vi "CursorShow.vi"(7 "nameShow":bool, 8 "错误输入（无错误）":errorcluster, 9 "游标.游标位置":T1, 10 "Type":T3 caption="事件类型", 11 "Graph":refnum<vi>) -> (0 "错误输出":errorcluster, 3 "引用输出":refnum<vi>)   [LabVIEW 2020]
uses:
  <vilib>/event_ctls.llb/lveventtype.ctl
  <vilib>/Utility/miscctls.llb/LVCursorListTypeDef.ctl
  <vilib>/Utility/miscctls.llb/LVPointDoubleTypeDef.ctl
panel:
  in  "游标列表":T2=[{"Name"="游标0", "Color"=16776960, "Style"=8, "Point Style"=13, "Name Visible"=TRUE, "Allow Drag"=TRUE, "Cursor Mode"=0, "Plot"=0, "Index"=0, "Position"={"X"=0.0, "Y"=0.0}, "X Scale"=0, "Y Scale"=0, "Watch Plots"=[], "Watch All Plots"=FALSE, "Plot Area"=0, "Label Offset"={"X"=0.0, "Y"=2.8391167192429023}}]
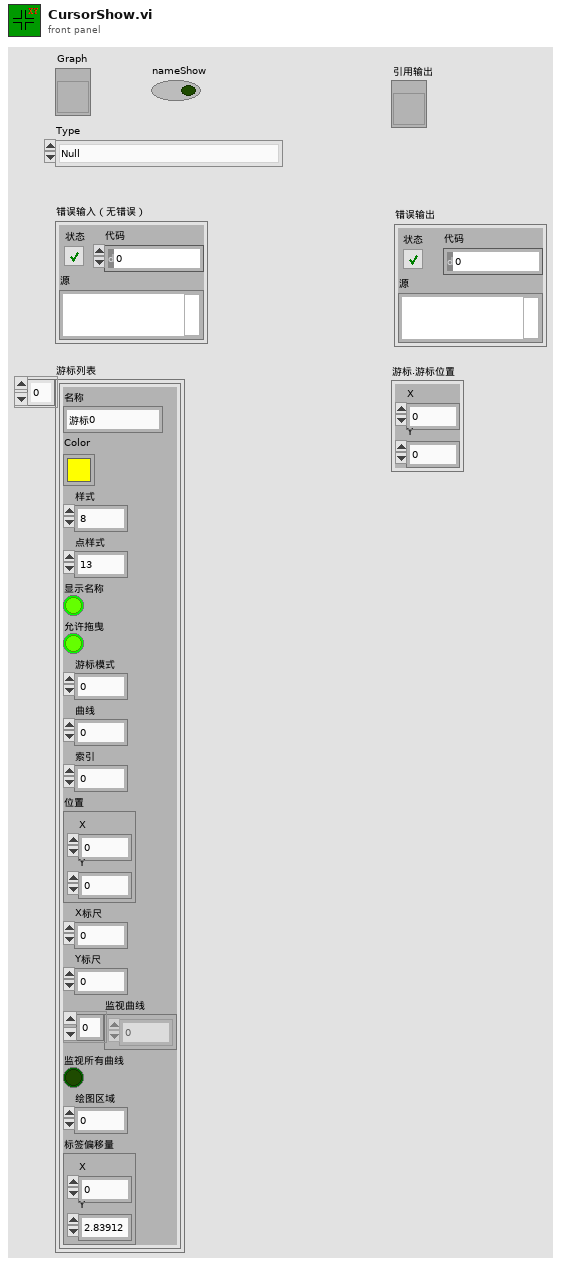
[diagram p1: front panel]
types:
  T1 = typedef "LVPointDoubleTypeDef.ctl" = cluster{"X":dbl, "Y":dbl}
  T2 = typedef "LVCursorListTypeDef.ctl" = cluster{"Name":string, "Color":u32, "Style":u8, "Point Style":u8, "Name Visible":bool, "Allow Drag":bool, "Cursor Mode":u32, "Plot":i32, "Index":i32, "Position":cluster{"X":dbl, "Y":dbl}, "X Scale":u32, "Y Scale":u32, "Watch Plots":i32[], "Watch All Plots":bool, "Plot Area":i32, "Label Offset":cluster{"X":dbl, "Y":dbl}}[]
  T3 = typedef "lveventtype.ctl" = enum32{"Null", "Timeout", "Annotation Menu Selection", "Annotation Menu Selection?", "App Instance Close", "App Instance Close?", "Autoscale Range Change", "Bookmark Info Change", "Cell Edit", "Cell Edit?", "Cursor Grab", "Cursor Grab?", "Cursor Menu Selection", "Cursor Menu Selection?", "Cursor Move", "Cursor Release", "Data Change", "Direction Change", "Display State Change", "Drag Ended", "Drag Enter", "Drag Leave", "Drag Over", "Drag Source Update", "Drag Starting", "Drag Starting?", "Drop", "Exec State Change", "Key Down", "Key Down?", "Key Repeat", "Key Repeat?", "Key Up", "Listbox Double Click", "Menu Activation?", "Menu Selection (App)", "Menu Selection? (App)", "Menu Selection (User)", "Mouse Down", "Mouse Down?", "Mouse Enter", "Mouse Leave", "Mouse Move", "Mouse Up", "Mouse Wheel", "NI Security User Change (App)", "Pane Size", "Panel Close", "Panel Close?", "Panel Resize", "Plot Attribute Change", "Scale Range Change", "Shortcut Menu Activation?", "Shortcut Menu Selection (App)", "Shortcut Menu Selection? (App)", "Shortcut Menu Selection (User)", "Tree Double Click", "Tree Drag", "Tree Drag?", "Tree Drop", "Tree Drop?", "Tree Item Close", "Tree Item Close?", "Tree Item Open", "Tree Item Open?", "User Event", "Value Change"}
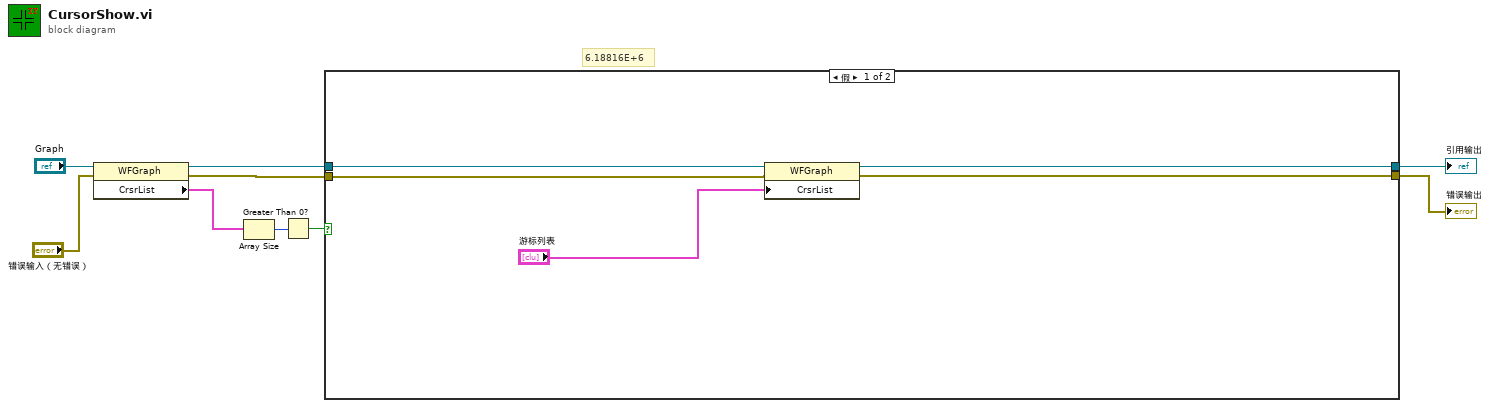
[diagram p0: block diagram]
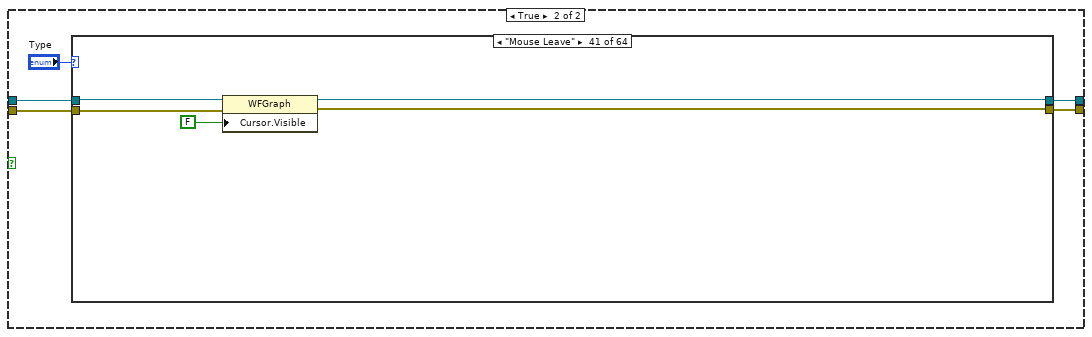
[diagram p2: hidden frame]
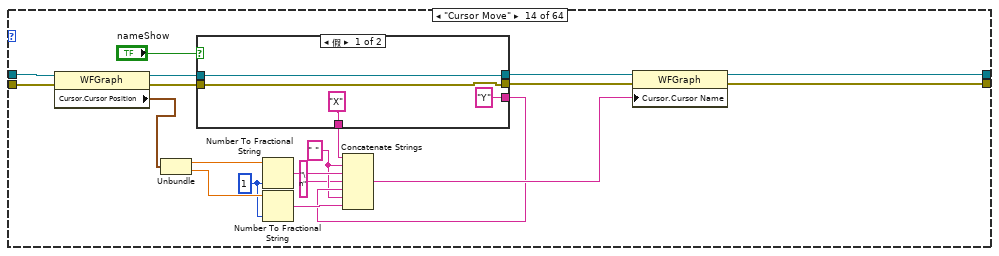
[diagram p16: hidden frame]
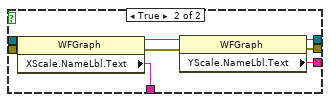
[diagram p17: hidden frame]
diagram:
  # "6.18816E+6"
  n1 = property class="WFGraph"(reference="Graph", error in="错误输入（无错误）") -> (reference out=w5:refnum<vi>, error out=w3:errorcluster, "CrsrList"=w8:T2)
  n2 = Array Size(array=w8) -> (size(s)=w9:i32)
  n3 = Greater Than 0?(x=w9) -> (x > 0?=w7:bool)
  n4 = case shown="假" w7 {
    tunnel: w5 -> [w14 w19]
    tunnel: w3 -> [w11 w17]
    tunnel: [w12 w16] -> w2
    tunnel: [w13 w15] -> w1
    frame False {
      n5 = property class="WFGraph"(reference=w14, error in=w11, "CrsrList"="游标列表") -> (reference out=w13:refnum<vi>, error out=w12:errorcluster)
    }
    frame True {
      n6 = case shown="\"Mouse Leave\"" "Type" {
        tunnel: w19 -> [_ _ _ _ _ _ _ _ _ _ _ _ _ w39 _ _ _ _ _ _ _ _ _ _ _ _ _ _ _ _ _ _ _ _ _ _ _ w54 _ w59 w66 _ _ _ _ _ _ _ _ _ _ _ _ _ _ _ _ _ _ _ _ _ _ _]
        tunnel: w17 -> [_ _ _ _ _ _ _ _ _ _ _ _ _ w25 _ _ _ _ _ _ _ _ _ _ _ _ _ _ _ _ _ _ _ _ _ _ _ _ _ w58 w64 _ _ _ _ _ _ _ _ _ _ _ _ _ _ _ _ _ _ _ _ _ _ _]
        tunnel: [_ _ _ _ _ _ _ _ _ _ _ _ _ w22 _ _ _ _ _ _ _ _ _ _ _ _ _ _ _ _ _ _ _ _ _ _ _ _ _ w56 w63 _ _ _ _ _ _ _ _ _ _ _ _ _ _ _ _ _ _ _ _ _ _ _] -> w16
        tunnel: [_ _ _ _ _ _ _ _ _ _ _ _ _ w21 _ _ _ _ _ _ _ _ _ _ _ _ _ _ _ _ _ _ _ _ _ _ _ w53 _ w55 w62 _ _ _ _ _ _ _ _ _ _ _ _ _ _ _ _ _ _ _ _ _ _ _] -> w15
        frame "Null", Default {
        }
        frame "Timeout" {
        }
        frame "Annotation Menu Selection" {
        }
        frame "Annotation Menu Selection?" {
        }
        frame "App Instance Close" {
        }
        frame "App Instance Close?" {
        }
        frame "Autoscale Range Change" {
        }
        frame "Cell Edit" {
        }
        frame "Cell Edit?" {
        }
        frame "Cursor Grab" {
        }
        frame "Cursor Grab?" {
        }
        frame "Cursor Menu Selection" {
        }
        frame "Cursor Menu Selection?" {
        }
        frame "Cursor Move" {
          w27 = " " ("字符串")
          w36 = i16 1 ("精度(6)")
          n7 = property class="WFGraph"(reference=w39, error in=w25) -> (reference out=w32:refnum<vi>, error out=w24:errorcluster, "Cursor.Cursor Position"=w34:T1)
          n8 = Unbundle(w34) -> ("Cursor X"=w38:dbl, "Cursor Y"=w37:dbl)
          n9 = case shown="假" "nameShow" {
            tunnel: w32 -> [w41 w51]
            tunnel: [w41 w49] -> w31
            tunnel: ["X" ("XScale.NameLbl.Text") w48] -> w30
            tunnel: ["Y" ("YScale.NameLbl.Text") w47] -> w28
            tunnel: w24 -> [w40 w46]
            tunnel: [w40 w44] -> w23
            frame False {
            }
            frame True {
              n10 = property class="WFGraph"(reference=w51, error in=w46) -> (reference out=w50:refnum<vi>, error out=w45:errorcluster, "XScale.NameLbl.Text"=w48:string)
              n11 = property class="WFGraph"(reference=w50, error in=w45) -> (reference out=w49:refnum<vi>, error out=w44:errorcluster, "YScale.NameLbl.Text"=w47:string)
            }
          }
          n12 = Number To Fractional String(number=w38, precision (6)=w36) -> (F-format string=w35:string)  [unwired: 2 in]
          n13 = Number To Fractional String(number=w37, precision (6)=w36) -> (F-format string=w29:string)  [unwired: 2 in]
          n14 = Concatenate Strings(w30, w27, w35, "\n" ("字符串"), w28, w27, w29) -> (w33:string)
          n15 = property class="WFGraph"(reference=w31, error in=w23, "Cursor.Cursor Name"=w33) -> (reference out=w21:refnum<vi>, error out=w22:errorcluster)
        }
        frame "Cursor Release" {
        }
        frame "Data Change" {
        }
        frame "Direction Change" {
        }
        frame "Display State Change" {
        }
        frame "Drag Ended" {
        }
        frame "Drag Enter" {
        }
        frame "Drag Leave" {
        }
        frame "Drag Over" {
        }
        frame "Drag Source Update" {
        }
        frame "Drag Starting" {
        }
        frame "Drag Starting?" {
        }
        frame "Drop" {
        }
        frame "Exec State Change" {
        }
        frame "Key Down" {
        }
        frame "Key Down?" {
        }
        frame "Key Repeat" {
        }
        frame "Key Repeat?" {
        }
        frame "Key Up" {
        }
        frame "Listbox Double Click" {
        }
        frame "Menu Activation?" {
        }
        frame "Menu Selection (App)" {
        }
        frame "Menu Selection? (App)" {
        }
        frame "Menu Selection (User)" {
        }
        frame "Mouse Down" {
          n16 = property class="WFGraph"(reference=w54, "Cursor.Cursor Position"="游标.游标位置") -> (reference out=w53:refnum<vi>)  [unwired: 1 in, 1 out]
        }
        frame "Mouse Down?" {
        }
        frame "Mouse Enter" {
          w61 = TRUE ("游标.可见")
          n17 = property class="WFGraph"(reference=w59, error in=w58, "Cursor.Visible"=w61) -> (reference out=w60:refnum<vi>, error out=w57:errorcluster)
          n18 = property class="WFGraph"(reference=w60, error in=w57, "Cursor.Cursor Name Visible"=w61) -> (reference out=w55:refnum<vi>, error out=w56:errorcluster)
        }
        frame "Mouse Leave" {
          n19 = property class="WFGraph"(reference=w66, error in=w64, "Cursor.Visible"=FALSE ("游标.可见")) -> (reference out=w62:refnum<vi>, error out=w63:errorcluster)
        }
        frame "Mouse Move" {
        }
        frame "Mouse Up" {
        }
        frame "NI Security User Change (App)" {
        }
        frame "Pane Size" {
        }
        frame "Panel Close" {
        }
        frame "Panel Close?" {
        }
        frame "Panel Resize" {
        }
        frame "Plot Attribute Change" {
        }
        frame "Scale Range Change" {
        }
        frame "Shortcut Menu Activation?" {
        }
        frame "Shortcut Menu Selection (App)" {
        }
        frame "Shortcut Menu Selection? (App)" {
        }
        frame "Shortcut Menu Selection (User)" {
        }
        frame "Tree Double Click" {
        }
        frame "Tree Drag" {
        }
        frame "Tree Drag?" {
        }
        frame "Tree Drop" {
        }
        frame "Tree Drop?" {
        }
        frame "Tree Item Close" {
        }
        frame "Tree Item Close?" {
        }
        frame "Tree Item Open" {
        }
        frame "Tree Item Open?" {
        }
        frame "Value Change" {
        }
      }
    }
  }
  "错误输出" <- w2
  "引用输出" <- w1
